vi "Start Data Listener.vi"(7 "Connection ID":u64, 8 "error in (no error)":errorcluster, 9 "Timeout (-1)":i32=-1, 10 "TCP  Ref":refnum<k5>, 11 "ConListenerQ":refnum<queue>) -> (0 "error out":errorcluster, 1 "timed out":bool)   [LabVIEW 2017, in "Front Panel Publisher.lvlib" / "Websocket.lvclass"]
doc: "Looks up an existing object matching object name or creates a new object and returns a refnum you can use when calling other class methods.\n\nObjects created with this VI should be destroyed using this class Delete VI."
uses:
  Websocket.lvclass
  Private/Connection Data.ctl
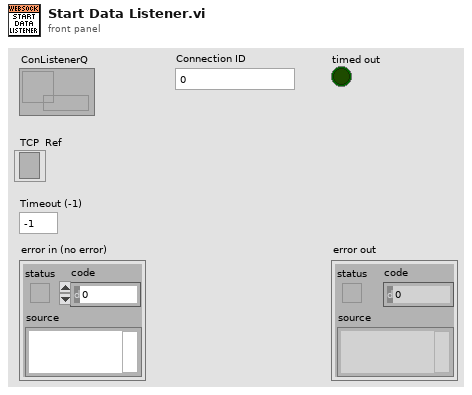
[diagram p1: front panel]
types:
  T1 = typedef "Front Panel Publisher.lvlib/Websocket.lvclass/Connection Data.ctl" = cluster{"TCP  Ref":refnum<k5>, "connection ID":u64, "ConListenerQ":refnum<queue>, "Page":string}
  T2 = enum16{"ReadRepository", "CreateNew", "CreateOrLookUpExisting", "ReadRepositoryAndDestroy"}
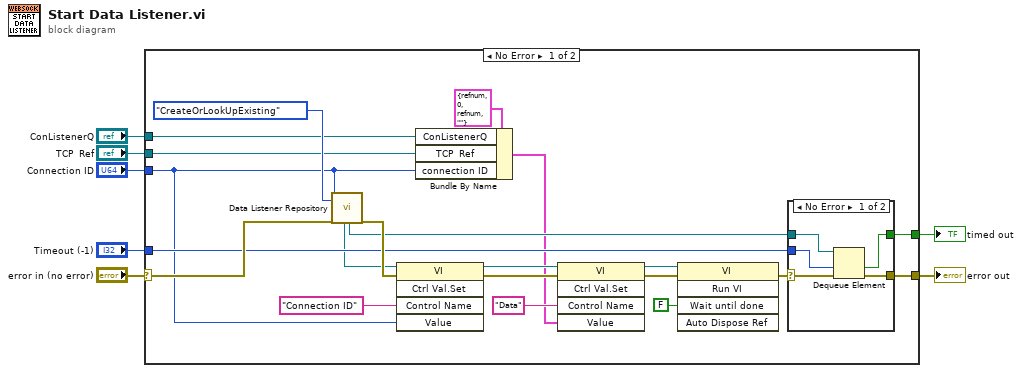
[diagram p0: block diagram]
diagram:
  n1 = case shown="No Error" "error in (no error)" {
    selector: "error in (no error)" -> [w27 w35]
    tunnel: [w28 w35] -> w6
    tunnel: "ConListenerQ" -> [w14 _]
    tunnel: "Timeout (-1)" -> [w24 _]
    tunnel: [w23 _] -> w3
    tunnel: "Connection ID" -> [w16 _]
    tunnel: "TCP  Ref" -> [w15 _]
    frame No Error {
      n2 = call "Data Listener Repository.vi"("Connection ID"=w16, "Action(ReadRepository)"=T2."CreateOrLookUpExisting", "error in (no error)"=w27) -> ("ProcessViRef"=w22:refnum<vi>, "ProcessSyncQueue"=w21:refnum<queue>, "error out"=w26:errorcluster)  [unwired: 11 in, 3 out]
      n3 = invoke class="VI" method="Ctrl Val.Set"(reference=w22, error in=w26, "Control Name"="Connection ID", "Value"=w16) -> (reference out=w13:refnum<vi>, error out=w12:errorcluster)  [unwired: 1 in, 3 out]
      n4 = Bundle By Name(cluster=T1 {"TCP  Ref"=refnum, "connection ID"=0, "ConListenerQ"=refnum, "Page"=""} ("Connection"), "ConListenerQ"=w14, "TCP  Ref"=w15, "connection ID"=w16) -> (w8:T1)
      n5 = invoke class="VI" method="Ctrl Val.Set"(reference=w13, error in=w12, "Control Name"="Data", "Value"=w8) -> (reference out=w10:refnum<vi>, error out=w11:errorcluster)  [unwired: 1 in, 3 out]
      n6 = invoke class="VI" method="Run VI"(reference=w10, error in=w11, "Wait until done"=FALSE ("Wait Until Done")) -> (error out=w25:errorcluster)  [unwired: 2 in, 4 out]
      n7 = case shown="No Error" w25 {
        tunnel: w21 -> [w31 _]
        tunnel: w24 -> [w30 _]
        tunnel: [w29 _] -> w23
        selector: w25 -> [w33 w34]
        tunnel: [w32 w34] -> w28
        frame No Error {
          n8 = Dequeue Element(queue=w31, timeout in ms (-1)=w30, error in (no error)=w33) -> (timed out?=w29:bool, error out=w32:errorcluster)  [unwired: 2 out]
        }
        frame Error {
        }
      }
    }
    frame Error {
    }
  }
  "error out" <- w6
  "timed out" <- w3
